vi "simple_control.vi"(8 "error in (no error)":errorcluster, 11 "Reactor to update":T2) -> (0 "Error out":errorcluster, 3 "Updated Reactor":T2)   [LabVIEW 2013]
uses:
  type_defs/reactor.ctl
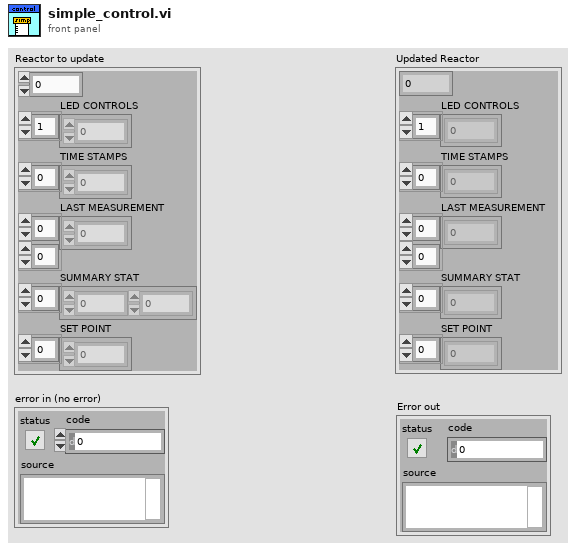
[diagram p1: front panel]
types:
  T1 = typedef "reactor.ctl" = dbl
  T2 = cluster{i32, "LED CONTROLS":dbl[], "TIME STAMPS":dbl[], "LAST MEASUREMENT":T1[][], "SUMMARY STAT":dbl[], "SET POINT":dbl[]}
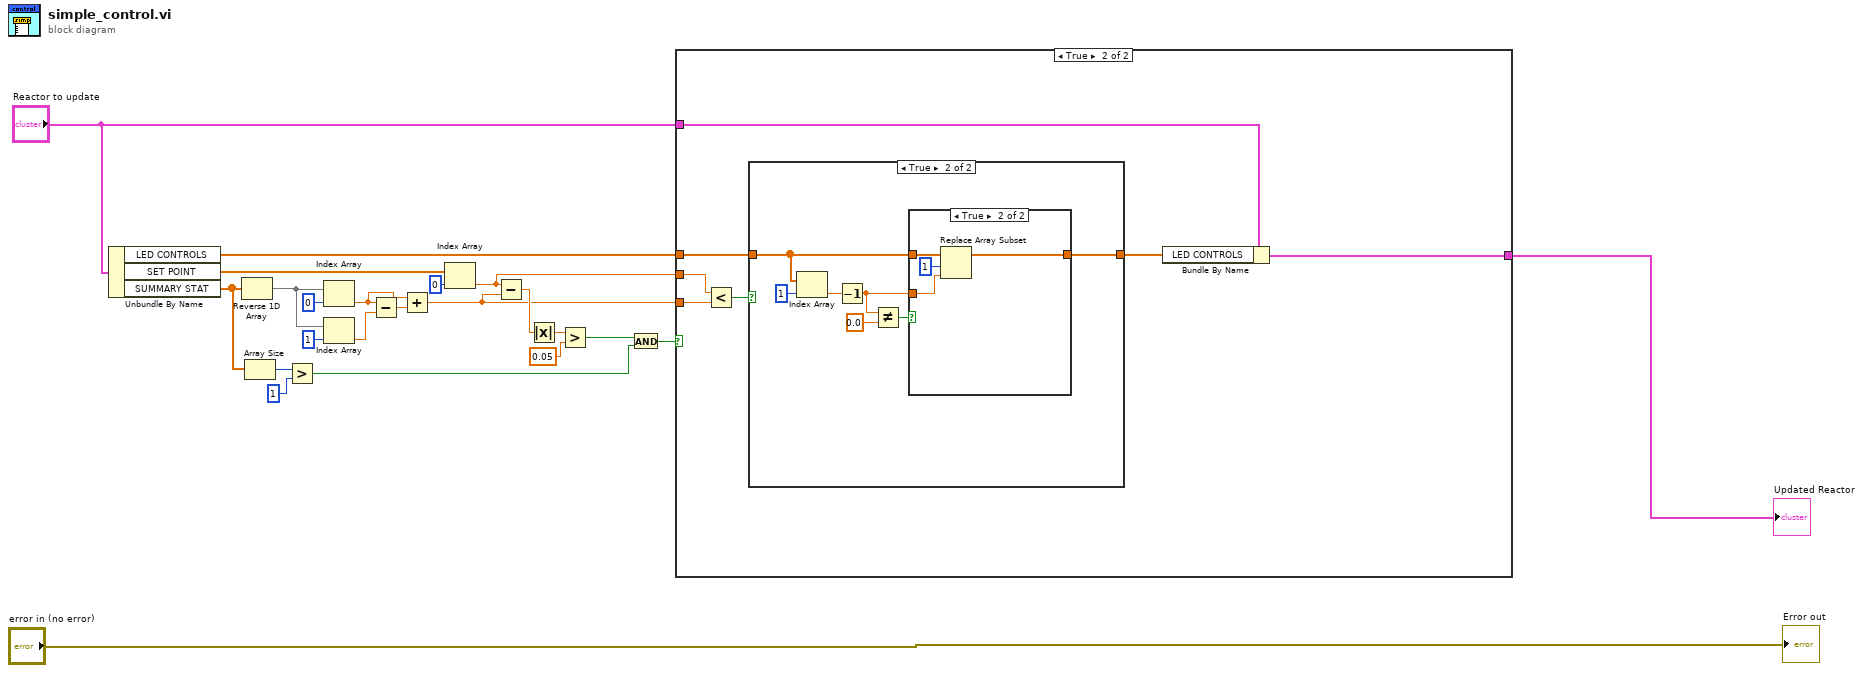
[diagram p0: block diagram]
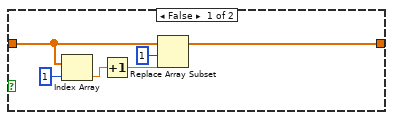
[diagram p3: hidden frame]
diagram:
  n1 = Unbundle By Name("Reactor to update") -> ("LED CONTROLS"=w18:dbl[], "SET POINT"=w13:dbl[], "SUMMARY STAT"=w6:dbl[])
  n2 = Reverse 1D Array(array=w6) -> (reversed array=w23:dbl[])
  n3 = Array Size(array=w6) -> (size(s)=w4:i32)
  n4 = Greater?(x=w4, y=1) -> (0:w2:bool)
  n5 = Index Array(array=w23, index=0) -> (element=w19:dbl)
  n6 = Index Array(array=w23, index=1) -> (element=w20:dbl)
  n7 = Subtract(x=w19, y=w20) -> (x-y=w14:dbl)
  n8 = Add(x=w19, y=w14) -> (x+y=w8:dbl)
  n9 = Index Array(array=w13, index=0) -> (element=w7:dbl)
  n10 = Subtract(x=w7, y=w8) -> (x-y=w9:dbl)
  n11 = Absolute Value(x=w9) -> (abs(x)=w11:dbl)
  n12 = Greater?(x=w11, y=0.05) -> (0:w5:bool)
  n13 = And(x=w5, y=w2) -> (x .and. y?=w1:bool)
  n14 = case shown="True" w1 {
    tunnel: w8 -> [_ w26]
    tunnel: w18 -> [_ w30]
    tunnel: "Reactor to update" -> [w24 w29]
    tunnel: [w24 w27] -> w16
    tunnel: w7 -> [_ w25]
    frame False {
    }
    frame True {
      n15 = Less?(x=w25, y=w26) -> (x < y?=w31:bool)
      n16 = case shown="True" w31 {
        tunnel: w30 -> [w37 w44]
        tunnel: [w32 w38] -> w28
        frame False {
          n17 = Index Array(array=w37, index=1) -> (element=w35:dbl)
          n18 = Increment(x=w35) -> (x+1=w34:dbl)
          n19 = Replace Array Subset(array=w37, new element=w34, index=1) -> (w32:dbl[])
        }
        frame True {
          n20 = Index Array(array=w44, index=1) -> (element=w43:dbl)
          n21 = Decrement(x=w43) -> (x-1=w40:dbl)
          n22 = Not Equal?(x=w40, y=0.0) -> (x != y?=w41:bool)
          n23 = case shown="True" w41 {
            tunnel: w44 -> [w45 w49]
            tunnel: w40 -> [_ w48]
            tunnel: [w45 w46] -> w38
            frame False {
            }
            frame True {
              n24 = Replace Array Subset(array=w49, new element=w48, index=1) -> (w46:dbl[])
            }
          }
        }
      }
      n25 = Bundle By Name(cluster=w29, "LED CONTROLS"=w28) -> (w27:T2)
    }
  }
  "Updated Reactor" <- w16
  "Error out" <- "error in (no error)"
